vi "DAC_manual_ramp_NI_ADC.vi"() -> ()   [LabVIEW 2013]
uses:
  <vilib>/DAQmx/read.llb/DAQmx Read (Analog 2D DBL NChan NSamp).vi
  <vilib>/DAQmx/create/channels.llb/DAQmx Create Channel (AI-Voltage-Basic).vi
  <vilib>/DAQmx/miscellaneous.llb/DAQmx Fill In Error Info.vi
  <resource>/objmgr/daqmx.rc
panel:
  in  "Save data":bool
  out "Ydata":dbl[][](array[numeric])
  out "Xdata":dbl[][](array[numeric])
  out "ADC values":dbl[](array[numeric])
  in  "DAC param":T1={"IP Adress FPGA"="192.168.1.21", "Delay(ms)"=1, "Busses to use"=[TRUE, TRUE, TRUE, TRUE, TRUE, TRUE, TRUE, TRUE], "max"=1.0, "min"=-1.0}
  in  "Clear graph":bool
  in  "ADC channel":dbl
  in  "Stop":bool
  in  "Go":bool
  in  "time per pt (ms)":dbl
  in  "Xparam":dbl
  out "XY Graph":cluster{dbl[], dbl[]}(graph)
  in  "Number of points":u32
  in  "Ramps":T2(array[cluster]) {"index" items=["0", "1", "2", "3", "4", "5", "6", "7"]; "bus" items=["0", "1", "2", "3", "4", "5", "6", "7"]}
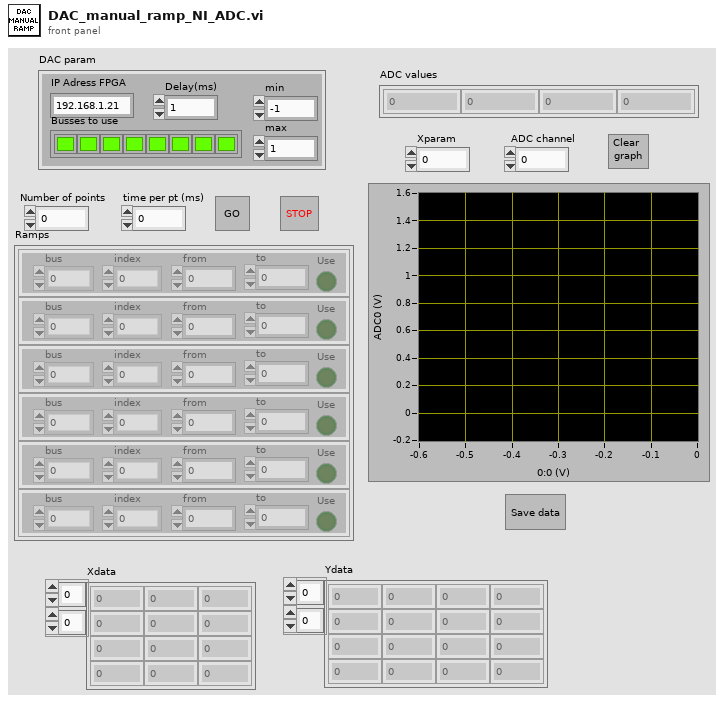
[diagram p1: front panel]
types:
  T1 = cluster{"IP Adress FPGA":string, "Delay(ms)":u8, "Busses to use":bool[], "max":dbl, "min":dbl}
  T2 = cluster{"bus":u16, "index":u16, "from":dbl, "to":dbl, "Use":bool}[]
  T3 = enum8{"start movement", "buses to use", "delay", "value", "stop", ""}
  T4 = cluster{"bus":u16, "index":u16, "from":dbl, "to":dbl, "Use":bool}
  T5 = typedef "fpga-bitfile-ref.ctl" = refnum<k20>
  T6 = enum8{"start movement", "buses to use", "delay", "value"}
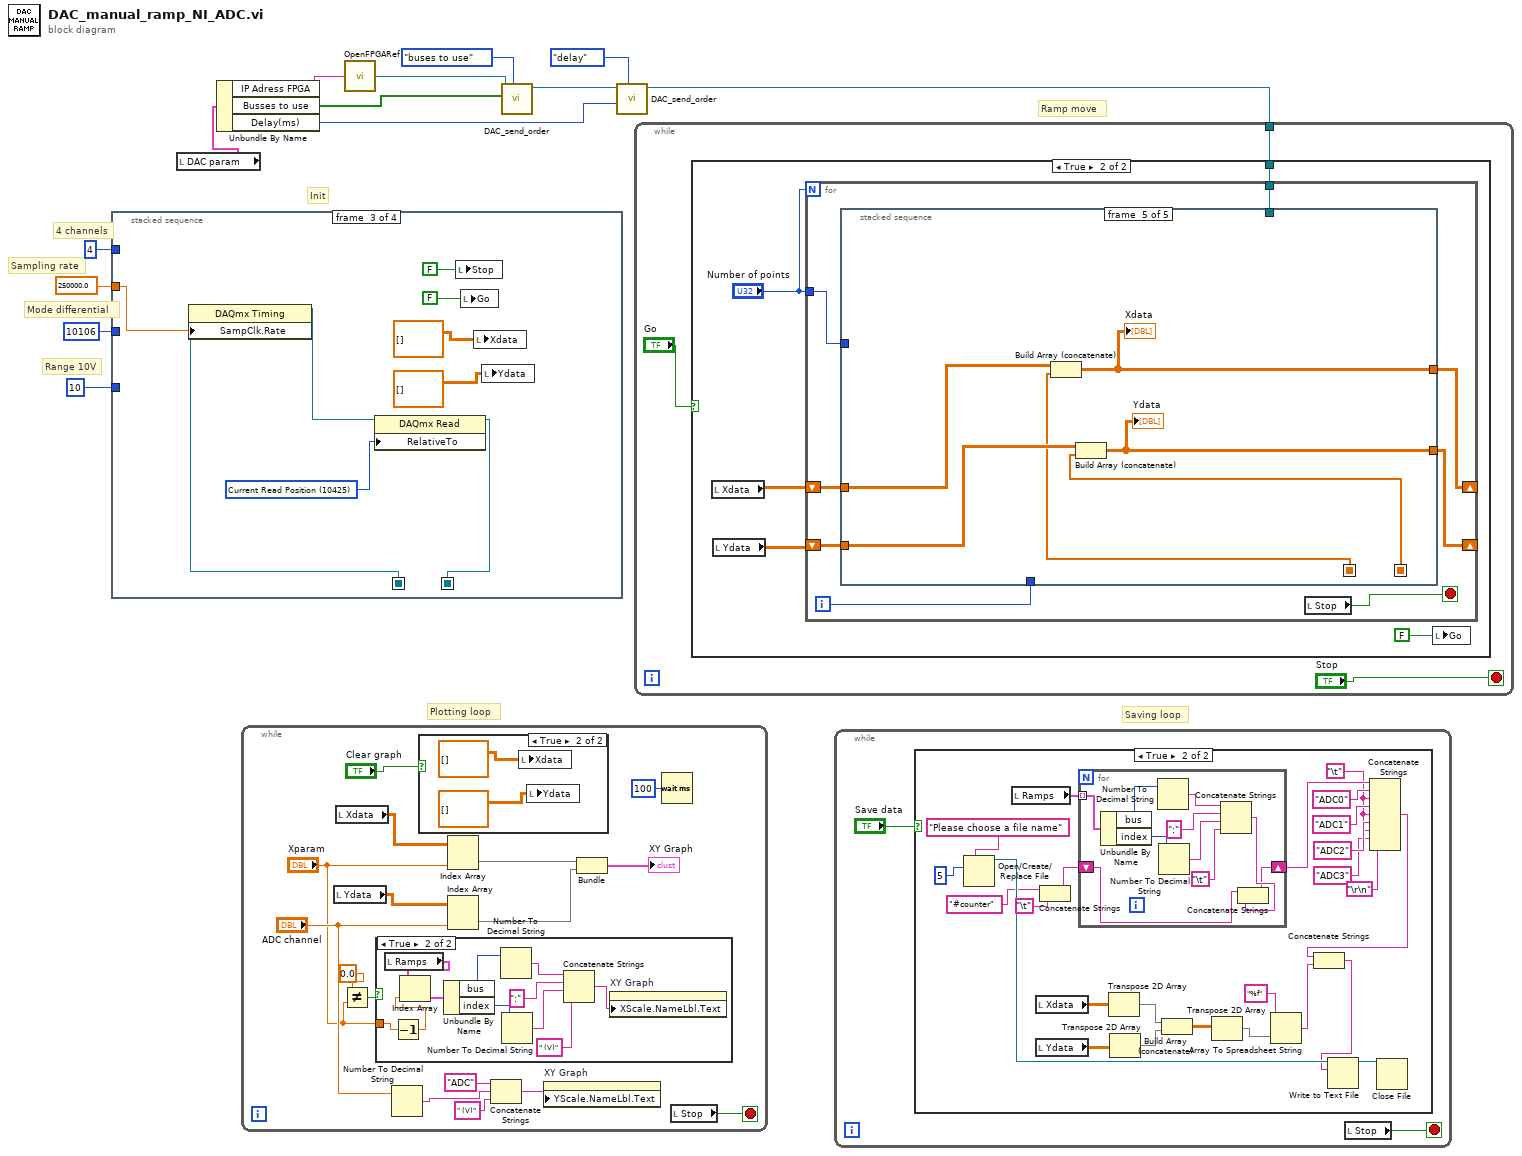
[diagram p0: block diagram]
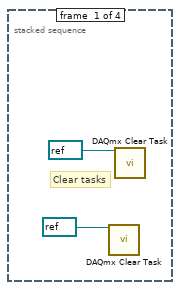
[diagram p2: hidden frame]
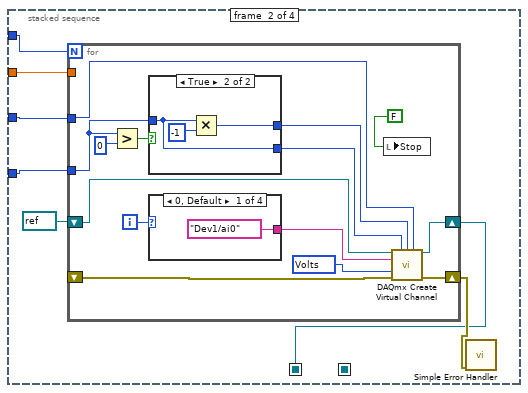
[diagram p3: hidden frame]
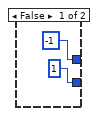
[diagram p4: hidden frame]
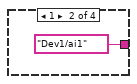
[diagram p5: hidden frame]
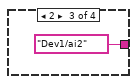
[diagram p6: hidden frame]
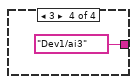
[diagram p7: hidden frame]
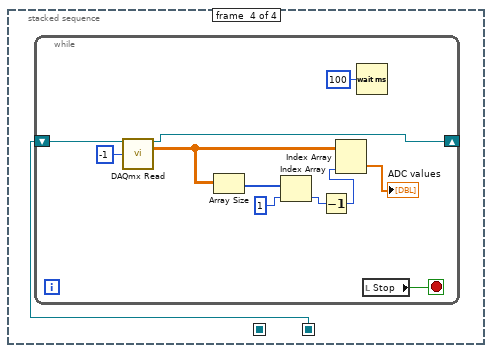
[diagram p8: hidden frame]
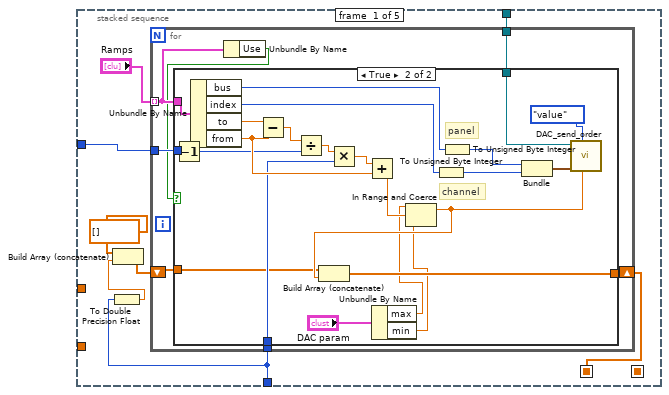
[diagram p10: hidden frame]
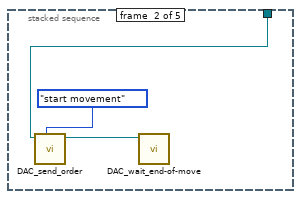
[diagram p12: hidden frame]
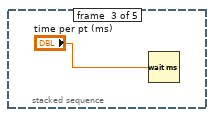
[diagram p13: hidden frame]
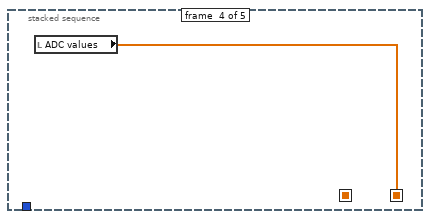
[diagram p14: hidden frame]
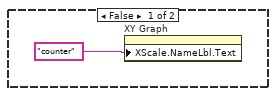
[diagram p17: hidden frame]
diagram:
  # "Init"
  # "Ramp move"
  # "Plotting loop"
  # "Saving loop"
  # "Sampling rate"
  # "Mode differential"
  # "Range 10V"
  # "4 channels"
  n1 = stacked-sequence {
    seq-local: [_ w16 _ _] -> [_ _ w53 _]
    seq-local: [_ _ w50 _] -> [_ _ _ w55]
    tunnel: 4 -> [_ w21 _ _]
    tunnel: 10106 -> [_ w20 _ _]
    tunnel: 10 -> [_ w19 _ _]
    tunnel: 250000.0 -> [_ w18 w54 _]
    frame #0 {
      # "Clear tasks"
      n2 = call <vilib>:"DAQmx Clear Task.vi"("task in"=refnum<k21> refnum ("task out in")) -> ()  [unwired: 14 in, 1 out]
      n3 = call <vilib>:"DAQmx Clear Task.vi"("task in"=refnum<k21> refnum ("task out in")) -> ()  [unwired: 14 in, 1 out]
    }
    frame #1 {
      n4 = for {
        N: w21 -> [_]
        shift-right: [w23] -> w16
        shift-left: refnum<k21> refnum ("task out") -> [w36]
        shift-right: [w33] -> w22
        shift-left: _ -> [w25]
        tunnel: w19 -> [w30]
        tunnel: w20 -> [w26]
        tunnel: w18 -> [_]
        i -> [w27]
        w34 = 10348 items=["Volts"=10348, "From Custom Scale"=10065] ("units")
        n5 = Greater?(x=w30, y=i16 0) -> (0:w31:bool)
        n6 = case shown="True" w31 {
          tunnel: w30 -> [_ w39]
          tunnel: [i16 -1 w40] -> w32
          tunnel: [i16 1 ("Range") w39] -> w28
          frame False {
          }
          frame True {
            n7 = Multiply(x=w39, y=i16 -1) -> (x*y=w40:i32)
          }
        }
        n8 = case shown="0, Default" w27 {
          tunnel: [tag "Dev1/ai0" ("physical channels") tag "Dev1/ai1" ("physical channels") tag "Dev1/ai2" ("physical channels") tag "Dev1/ai3" ("physical channels")] -> w35
          frame 0, Default {
          }
          frame 1 {
          }
          frame 2 {
          }
          frame 3 {
          }
        }
        n9 = local write "Stop"(FALSE) -> ()
        n10 = call-poly <vilib>:"DAQmx Create Virtual Channel.vi"("task in"=w36, "maximum value"=w28, "minimum value"=w32, "input terminal configuration"=w26, "physical channels"=w35, "units"=w34, "error in"=w25) -> ("task out"=w23:refnum<k21>, "error out"=w33:errorcluster)  [unwired: 2 in, 5 out]
      }
      n11 = call <vilib>:"Simple Error Handler.vi"("error in (no error)"=w22) -> ()  [unwired: 4 in, 5 out]
    }
    frame #2 {
      w52 = 10425 items=["First Sample"=10424, "Current Read Position"=10425, "Reference Trigger"=10426, "First Pretrigger Sample"=10427, "Most Recent Sample"=10428] ("RelativeTo")
      n12 = property class="DAQmx Timing"(reference=w53, "SampClk.Rate"=w54) -> (reference out=w51:refnum<k21>)  [unwired: 1 in, 1 out]
      n13 = property class="DAQmx Read"(reference=w51, "RelativeTo"=w52) -> (reference out=w50:refnum<k21>)  [unwired: 1 in, 1 out]
      n14 = local write "Stop"(FALSE) -> ()
      n15 = local write "Go"(FALSE) -> ()
      n16 = local write "Xdata"(dbl[][] []) -> ()
      n17 = local write "Ydata"(dbl[][] []) -> ()
    }
    frame #3 {
      n18 = while {
        shift-right: [w60] -> _
        shift-left: w55 -> [w61]
        stop <- w66 stop-if-true
        n19 = call-poly <vilib>:"DAQmx Read.vi"("task/channels in"=w61, "number of samples per channel"=-1) -> ("task out"=w60:refnum<k21>, "data"=w63:dbl[][])  [unwired: 11 in, 1 out]
        n20 = Array Size(array=w63) -> (size(s)=w64:i32[])
        n21 = Index Array(array=w64, index=1) -> (element=w57:i32)
        n22 = Decrement(x=w57) -> (x-1=w56:i32)
        n23 = Index Array(array=w63, index (col)=w56) -> (element=→"ADC values":dbl[])  [unwired: 1 in]
        n24 = Wait (ms)(milliseconds to wait=100) -> ()  [unwired: 1 out]
        n25 = local read "Stop"() -> (w66:bool)
      }
    }
  }
  n26 = local read "DAC param"() -> (w3:T1)
  n27 = Unbundle By Name(w3) -> ("IP Adress FPGA"=w6:string, "Busses to use"=w5:bool[], "Delay(ms)"=w4:u8)
  n28 = while {
    stop <- w80 stop-if-true
    n29 = local read "Ydata"() -> (w78:dbl[][])
    n30 = local read "Xdata"() -> (w79:dbl[][])
    n31 = Not Equal?(x=0.0, y="Xparam") -> (x != y?=w70:bool)
    n32 = case shown="True" w70 {
      tunnel: "Xparam" -> [_ w87]
      frame False {
        n33 = property on="XY Graph" class="XYGraph (strict)"("XScale.NameLbl.Text"="counter") -> ()  [unwired: 2 in, 2 out]
      }
      frame True {
        n34 = local read "Ramps"() -> (w96:T2)
        n35 = Decrement(x=w87) -> (x-1=w86:dbl)
        n36 = Index Array(array=w96, index=w86) -> (element=w95:T4)
        n37 = Unbundle By Name(w95) -> ("bus"=w94:u16, "index"=w93:u16)
        n38 = Number To Decimal String(number=w94) -> (decimal integer string=w91:string)  [unwired: 1 in]
        n39 = Number To Decimal String(number=w93) -> (decimal integer string=w92:string)  [unwired: 1 in]
        n40 = Concatenate Strings(w91, ":", w92, " (V)") -> (w88:string)
        n41 = property on="XY Graph" class="XYGraph (strict)"("XScale.NameLbl.Text"=w88) -> ()  [unwired: 2 in, 2 out]
      }
    }
    n42 = Number To Decimal String(number="ADC channel") -> (decimal integer string=w72:string)  [unwired: 1 in]
    n43 = case shown="True" "Clear graph" {
      frame False {
      }
      frame True {
        n44 = local write "Xdata"(dbl[][] []) -> ()
        n45 = local write "Ydata"(dbl[][] []) -> ()
      }
    }
    n46 = Index Array(array=w79, index (col)="Xparam") -> (element=w81:dbl[])  [unwired: 1 in]
    n47 = Index Array(array=w78, index (col)="ADC channel") -> (element=w82:dbl[])  [unwired: 1 in]
    n48 = Concatenate Strings("ADC", w72, " (V)") -> (w73:string)
    n49 = property on="XY Graph" class="XYGraph (strict)"("YScale.NameLbl.Text"=w73) -> ()  [unwired: 2 in, 2 out]
    n50 = Bundle("Xdata"=w81, "Ydata"=w82) -> (→"XY Graph":cluster{"Xdata":dbl[], "Ydata":dbl[]})  [unwired: 1 in]
    n51 = Wait (ms)(milliseconds to wait=100) -> ()  [unwired: 1 out]
    n52 = local read "Stop"() -> (w80:bool)
  }
  n53 = call "OpenFPGARef.vi"("IP Address"=w6) -> ("FPGA VI Reference Out"=w7:T5)
  n54 = call "DAC_send_order.vi"("order"=T3."buses to use", "buses to use"=w5, "FPGA VI Reference In"=w7) -> ("FPGA VI Reference Out"=w8:T5)  [unwired: 8 in]
  n55 = call "DAC_send_order.vi"("order"=T3."delay", "delay between steps (ms)"=w4, "FPGA VI Reference In"=w8) -> ("FPGA VI Reference Out"=w2:T5)  [unwired: 8 in]
  n56 = while {
    tunnel: w2 -> [w98]
    stop <- "Stop" stop-if-true
    n57 = case shown="True" "Go" {
      tunnel: w98 -> [_ w104]
      frame False {
      }
      frame True {
        n58 = local read "Xdata"() -> (w102:dbl[][])
        n59 = local read "Ydata"() -> (w101:dbl[][])
        n60 = for {
          N: "Number of points" -> [_]
          tunnel: "Number of points" -> [w112]
          tunnel: w104 -> [w111]
          shift-right: [w106] -> _
          shift-left: w102 -> [w109]
          shift-right: [w107] -> _
          shift-left: w101 -> [w108]
          i -> [w110]
          stop <- w105 stop-if-true
          n61 = stacked-sequence {
            seq-local: [w118 _ _ _ _] -> [_ _ _ _ w159]
            seq-local: [_ _ _ w156 _] -> [_ _ _ _ w162]
            tunnel: w112 -> [w120 _ _ _ _]
            tunnel: w111 -> [w119 w154 _ _ _]
            tunnel: [_ _ _ _ w158] -> w106
            tunnel: [_ _ _ _ w157] -> w107
            tunnel: w110 -> [w116 _ _ _ _]
            tunnel: w109 -> [_ _ _ _ w161]
            tunnel: w108 -> [_ _ _ _ w160]
            frame #0 {
              n62 = To Double Precision Float(number=w116) -> (double precision float=w114:dbl)
              n63 = Build Array (concatenate)(dbl[] [], w114) -> (w113:dbl[])
              n64 = for {
                tunnel: "Ramps" -> [w122] mode=indexing
                tunnel: w120 -> [w127]
                tunnel: w119 -> [w126]
                shift-right: [w125] -> w118
                shift-left: w113 -> [w124]
                tunnel: w116 -> [w123]
                n65 = Unbundle By Name(w122) -> ("Use"=w121:bool)
                n66 = case shown="True" w121 {
                  tunnel: w122 -> [_ w151]
                  tunnel: w127 -> [_ w145]
                  tunnel: w126 -> [_ w139]
                  tunnel: [w128 w135] -> w125
                  tunnel: w124 -> [w128 w129]
                  tunnel: w123 -> [_ w134]
                  frame False {
                  }
                  frame True {
                    # "channel"
                    # "panel"
                    n67 = Decrement(x=w145) -> (x-1=w144:u32)
                    n68 = Unbundle By Name(w151) -> ("bus"=w138:u16, "index"=w137:u16, "to"=w150:dbl, "from"=w146:dbl)
                    n69 = Subtract(x=w150, y=w146) -> (x-y=w149:dbl)
                    n70 = Divide(x=w149, y=w144) -> (x/y=w148:dbl)
                    n71 = Multiply(x=w148, y=w134) -> (x*y=w147:dbl)
                    n72 = Add(x=w147, y=w146) -> (x+y=w132:dbl)
                    n73 = Unbundle By Name("DAC param") -> ("max"=w131:dbl, "min"=w130:dbl)
                    n74 = In Range and Coerce(upper limit=w131, x=w132, lower limit=w130) -> (coerced(x)=w136:dbl)  [unwired: 1 out]
                    n75 = Build Array (concatenate)(w129, w136) -> (w135:dbl[])
                    n76 = To Unsigned Byte Integer(number=w137) -> (unsigned 8bit integer=w141:u8)
                    n77 = To Unsigned Byte Integer(number=w138) -> (unsigned 8bit integer=w142:u8)
                    n78 = Bundle(w142, w141) -> (w140:cluster{u8, u8})  [unwired: 1 in]
                    n79 = call "DAC_send_order.vi"("DAC goto value"=w136, "order"=T6."value", "Cluster"=w140, "FPGA VI Reference In"=w139) -> ()  [unwired: 3 in, 5 out]
                  }
                }
              }
            }
            frame #1 {
              n80 = call "DAC_send_order.vi"("order"=T6."start movement", "FPGA VI Reference In"=w154) -> ("FPGA VI Reference Out"=w152:T5)  [unwired: 5 in, 4 out]
              n81 = call "DAC_wait_end-of-move.vi"("FPGA VI Reference In"=w152) -> ()  [unwired: 10 in, 1 out]
            }
            frame #2 {
              n82 = Wait (ms)(milliseconds to wait="time per pt (ms)") -> ()  [unwired: 1 out]
            }
            frame #3 {
              n83 = local read "ADC values"() -> (w156:dbl[])
            }
            frame #4 {
              n84 = Build Array (concatenate)(w161, w159) -> (w158:dbl[][])
              "Xdata" <- w158
              n85 = Build Array (concatenate)(w160, w162) -> (w157:dbl[][])
              "Ydata" <- w157
            }
          }
          n86 = local read "Stop"() -> (w105:bool)
        }
        n87 = local write "Go"(FALSE) -> ()
      }
    }
  }
  n88 = while {
    stop <- w163 stop-if-true
    n89 = case shown="True" "Save data" {
      frame False {
      }
      frame True {
        w173 = "\t"
        n90 = Open/Create/Replace File(prompt="Please choose a file name", operation (0:open)=5) -> (refnum out=w172:refnum<file>)  [unwired: 4 in, 2 out]
        n91 = local read "Ramps"() -> (w180:T2)
        n92 = local read "Xdata"() -> (w187:dbl[][])
        n93 = local read "Ydata"() -> (w186:dbl[][])
        n94 = Concatenate Strings("#counter", "\t") -> (w166:string)
        n95 = for {
          tunnel: w180 -> [w194] mode=indexing
          shift-right: [w191] -> w179
          shift-left: w166 -> [w193]
          n96 = Unbundle By Name(w194) -> ("bus"=w195:u16, "index"=w196:u16)
          n97 = Number To Decimal String(number=w195) -> (decimal integer string=w198:string)  [unwired: 1 in]
          n98 = Number To Decimal String(number=w196) -> (decimal integer string=w197:string)  [unwired: 1 in]
          n99 = Concatenate Strings(w198, ":", w197, "\t") -> (w192:string)
          n100 = Concatenate Strings(w193, w192) -> (w191:string)
        }
        n101 = Transpose 2D Array(2D array=w187) -> (transposed array=w185:dbl[][])
        n102 = Transpose 2D Array(2D array=w186) -> (transposed array=w184:dbl[][])
        n103 = Build Array (concatenate)(w185, w184) -> (w183:dbl[][])
        n104 = Transpose 2D Array(2D array=w183) -> (transposed array=w182:dbl[][])
        n105 = Array To Spreadsheet String(array=w182, 3:"%f") -> (spreadsheet string=w170:string)  [unwired: 1 in]
        n106 = Concatenate Strings(w179, "ADC0", w173, "ADC1", w173, "ADC2", w173, "ADC3", "\r\n") -> (w171:string)
        n107 = Concatenate Strings(w171, w170) -> (w169:string)
        n108 = Write to Text File(file (use dialog)=w172, text=w169) -> (refnum out=w165:refnum<file>)  [unwired: 2 in, 2 out]
        n109 = Close File(refnum=w165) -> ()  [unwired: 1 in, 2 out]
      }
    }
    n110 = local read "Stop"() -> (w163:bool)
  }
